vi "SynchronousAPI_TEMPLATE.vi"(6 "timeout (50 ms)":i32=50, 8 "error in (no error)":errorcluster, 10 "myData":string, 11 "SMO.jsonRPC":refnum<class "SMO.jsonRPC.lvclass">) -> (0 "error out":errorcluster, 1 "id":i32, 2 "reply":string, 3 "SMO.jsonRPC out":refnum<class "SMO.jsonRPC.lvclass">)   [LabVIEW 2013, in "SMO.jsonRPC.lvclass"]
doc: "---------------------------------------------------------------\nJKI State Machine Objects™\nhttp://jki.net/state-machine-objects/\nCopyright (C) 2005-2015, JKI <info@jki.net>\nALL RIGHTS RESERVEDJKI State Machine Objects (SMO) 1.0.0.5\nJKI - JKI\nCopyright (c) 2016, JKI"
uses:
  SMO.jsonRPC.lvclass
panel:
  # "For instructions on how to use the JKI State Machine Objects, examples and video tutorials, visit:\nhttp://jki.net/state-machine-objects/\n\nJKI State Machine Objects™\nhttp://jki.net/state-machine-objects/\nCopyright (C) 2005-2015, JKI <info@jki.net>\nALL RIGHTS RESERVED"
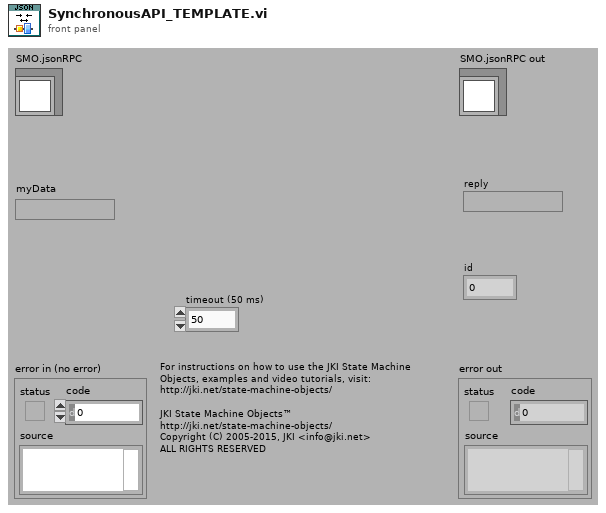
[diagram p1: front panel]
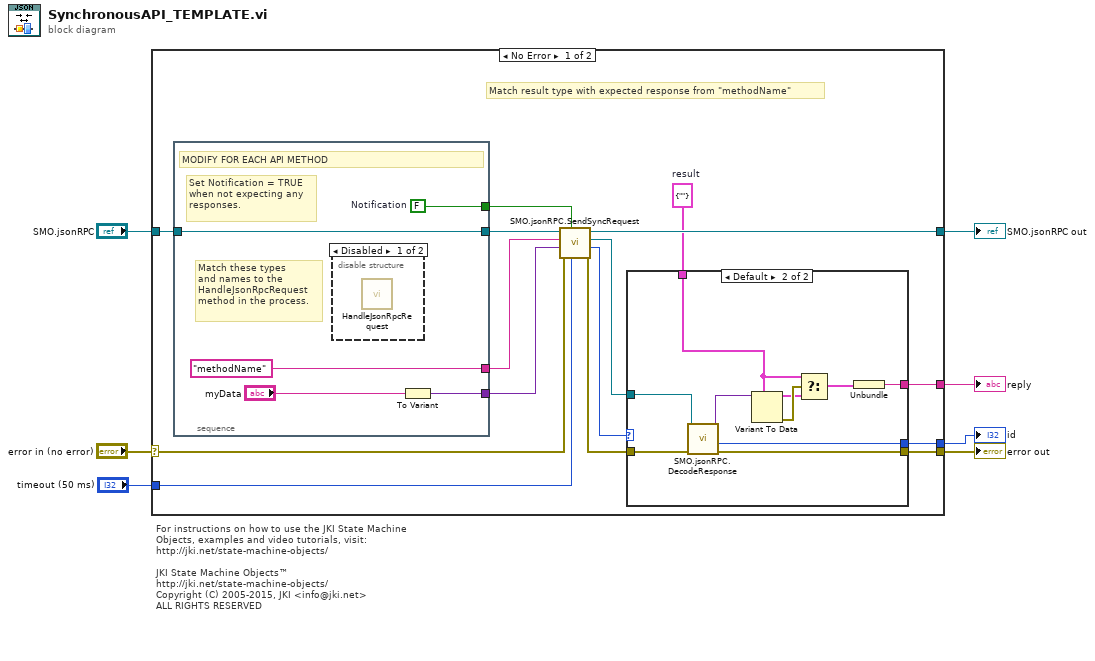
[diagram p0: block diagram]
diagram:
  # "For instructions on how to use the JKI State Machine Objects, examples and video tutorials, visit:\nhttp://jki.net/state-machine-objects/\n\nJKI State Machine Objects™\nhttp://jki.net/state-machine-objects/\nCopyright (C) 2005-2015, JKI <info@jki.net>\nALL RIGHTS RESERVED"
  n1 = case shown="No Error" "error in (no error)" {
    selector: "error in (no error)" -> [w21 w40]
    tunnel: "SMO.jsonRPC" -> [w15 w41]
    tunnel: [w22 w41] -> w6
    tunnel: "timeout (50 ms)" -> [w12 _]
    tunnel: [w19 _] -> w3
    tunnel: [w11 _] -> w2
    tunnel: [w13 w40] -> w1
    frame No Error {
      w9 = cluster{string} {""}  # result
      # "Match result type with expected response from \"methodName\""
      n2 = stacked-sequence {
        tunnel: ["methodName" ("Method")] -> w18
        tunnel: [w36] -> w17
        tunnel: [w37] -> w16
        tunnel: w15 -> [w37]
        tunnel: [w35] -> w10
        frame #0 {
          w35 = FALSE  # Notification
          # "Set Notification = TRUE\nwhen not expecting any\nresponses."
          # "Match these types\nand names to the\nHandleJsonRpcRequest\nmethod in the process."
          # "MODIFY FOR EACH API METHOD"
          n3 = disable-structure shown="Disabled" {
            frame Disabled {
              n4 = call "HandleJsonRpcRequest.vi"() -> ()  [unwired: 9 in, 3 out]
            }
            frame Enabled {
            }
          }
          n5 = To Variant(anything="myData") -> (Variant=w36:variant)
        }
      }
      n6 = call "SMO.jsonRPC.SendSyncRequest.vi"("timeout (50ms)"=w12, "Notification (F)"=w10, "error in (no error)"=w21, "Parameters"=w17, "Method"=w18, "SMO.jsonRPC in"=w16) -> ("error out"=w14:errorcluster, "id"=w8:i32, "Response"=w20:refnum<class "Response.lvclass">, "SMO.jsonRPC out"=w22:refnum<class "SMO.jsonRPC.lvclass">)  [unwired: 2 in]
      n7 = case shown="Default" w8 {
        selector: w8 -> [w23 _]
        tunnel: w20 -> [_ w26]
        tunnel: [_ w34] -> w19
        tunnel: w14 -> [w24 w29]
        tunnel: [w24 w28] -> w13
        tunnel: [w23 w27] -> w11
        tunnel: w9 -> [_ w30]
        frame -1 {
          # "Notification\n==============\nNo response expected."
        }
        frame Default {
          n8 = call "SMO.jsonRPC.DecodeResponse.vi"("error in (no error)"=w29, "jsonRPC response"=w26) -> ("error out"=w28:errorcluster, "id"=w27:i32, "result"=w25:variant)  [unwired: 7 in]
          n9 = Variant To Data(type=w30, Variant=w25) -> (data=w32:cluster{string}, error out=w33:errorcluster)  [unwired: 1 in]
          n10 = Select(t=w30, s=w33, f=w32) -> (s? t:f=w31:cluster{string})
          n11 = Unbundle(w31) -> (w34:string)
        }
      }
    }
    frame Error {
    }
  }
  "error out" <- w1
  "SMO.jsonRPC out" <- w6
  "reply" <- w3
  "id" <- w2
